vi "Filter SRs.vi"(8 "error in":errorcluster, 9 "Legend":refnum<vi>, 10 "Filter Cluster":T1={"Show Resolved"=TRUE, "Show Potentially Resolved"=TRUE, "Show Passoffs"=TRUE, "Show In Collab"=TRUE}, 11 "list in":T2[](array[typedef]) {"Creation Date" format="%<%x>T"; "Last Updated" format="%<%x>T"}) -> (0 "error out":errorcluster, 3 "list out":T2[](array[typedef]) {"Creation Date" format="%<%x>T"; "Last Updated" format="%<%x>T"})   [LabVIEW 2018]
uses:
  Type Defs/SR Cluster.ctl
  Type Defs/SR Status.ctl
  Type Defs/Filter Cluster.ctl
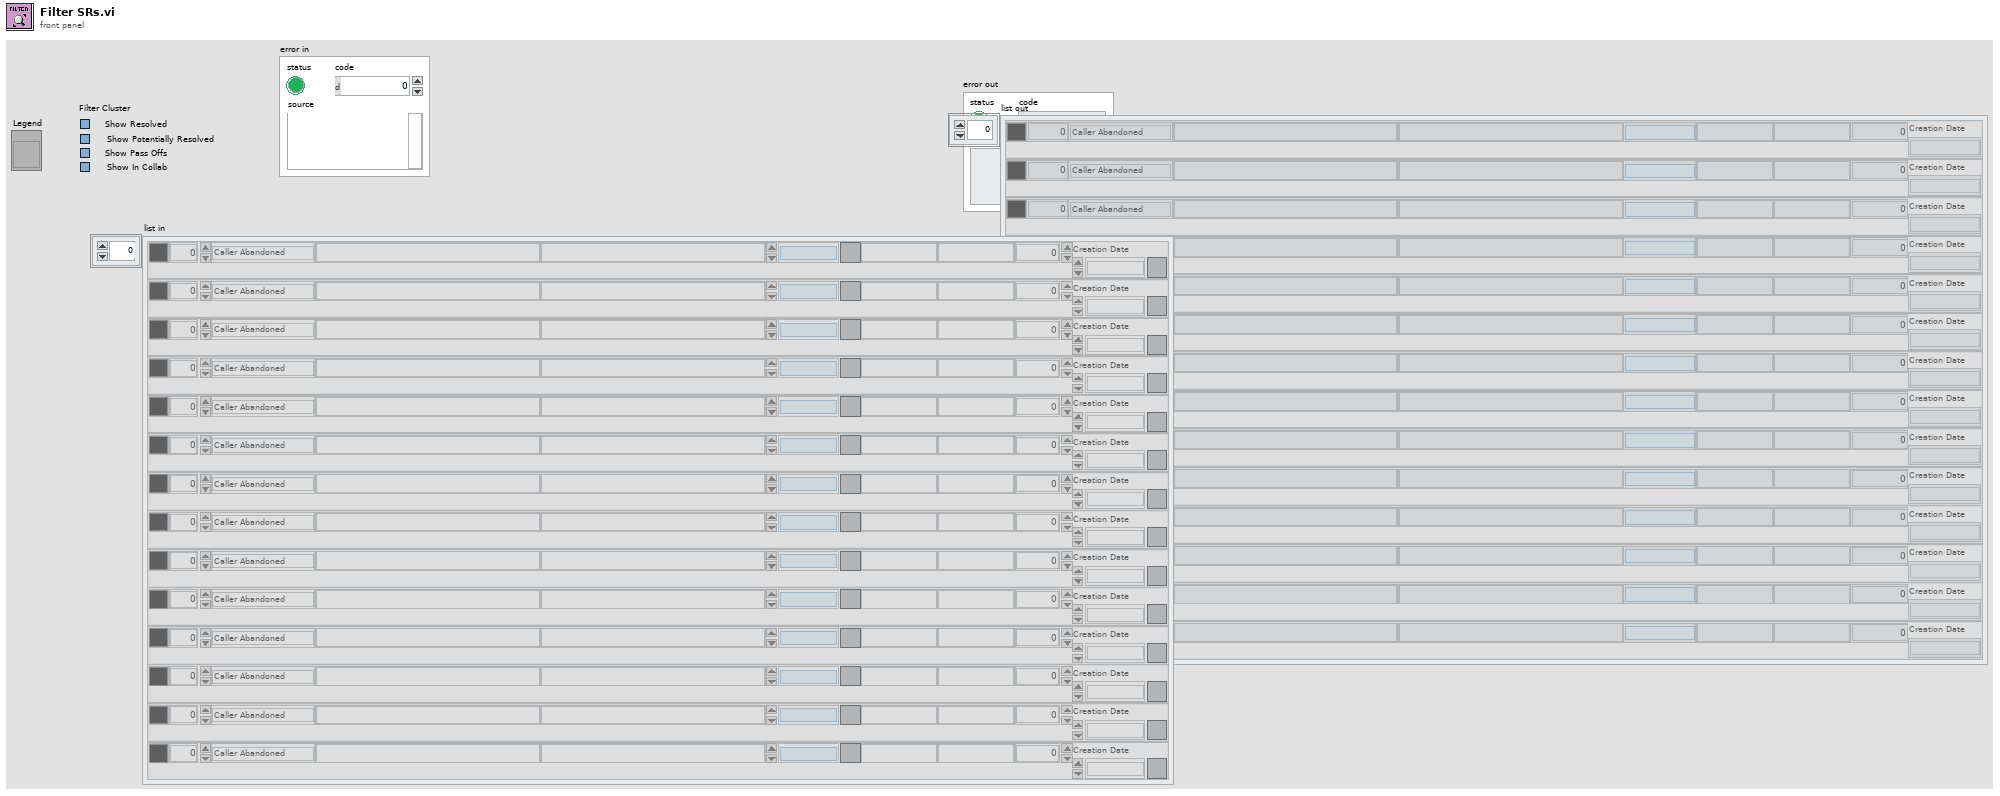
[diagram p1: front panel]
types:
  T1 = typedef "Filter Cluster.ctl" = cluster{"Show Resolved":bool, "Show Potentially Resolved":bool, "Show Passoffs":bool, "Show In Collab":bool}
  T2 = typedef "SR Cluster.ctl" = cluster{"Color":u32, "SR Number":i32, "SR Status":T3, "Name":string, "Summary":string, "Last Updated":timestamp, "SR Type":string, "Service Level":string, "Days Open":dbl, "Creation Date":timestamp}
  T3 = typedef "SR Status.ctl" = enum16{"Caller Abandoned", "Created in Error", "Expired", "Forum Resolved AE", "Forum Resolved Customer", "IN WORK", "IN WORK Collab with AES", "IN WORK Collab with PSE", "IN WORK Collab with SE", "IN WORK Customer Added Note", "IN WORK Escalation", "IN WORK Wait on Customer", "Open", "Potentially Resolved", "Presumed Resolved", "RMA Approved for Return", "RMA Closed", "RMA Closed - DOA", "RMA In Progress", "RMA Open", "RMA Waiting on Customer", "Resolved", "Passed Off"}
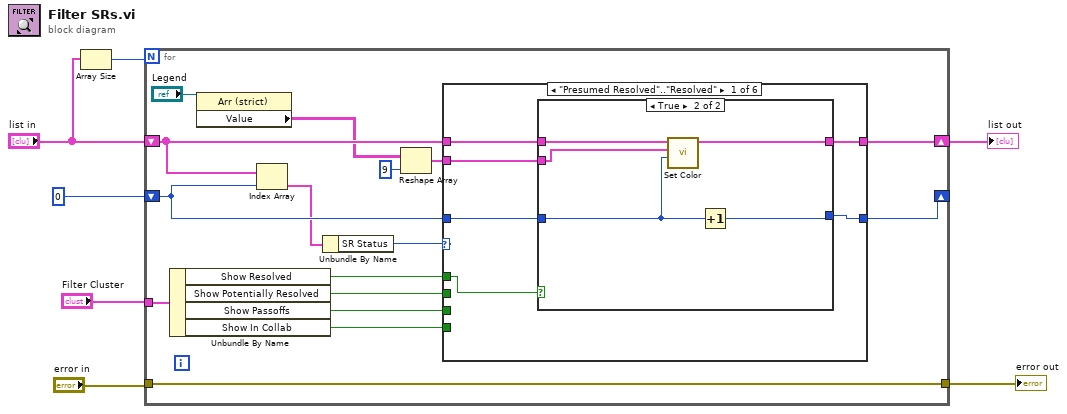
[diagram p0: block diagram]
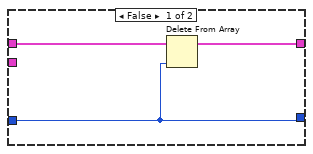
[diagram p2: hidden frame]
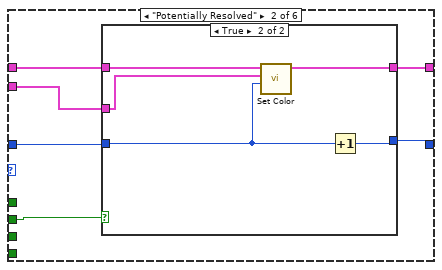
[diagram p3: hidden frame]
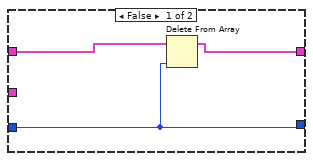
[diagram p4: hidden frame]
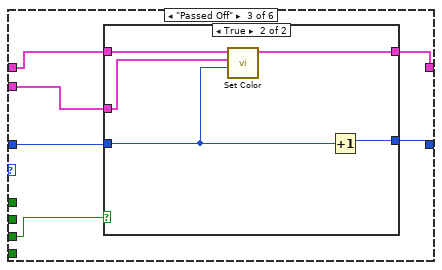
[diagram p5: hidden frame]
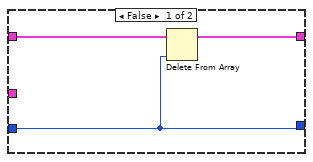
[diagram p6: hidden frame]
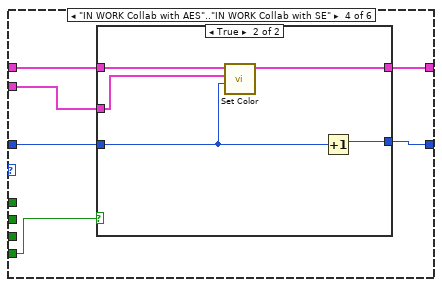
[diagram p7: hidden frame]
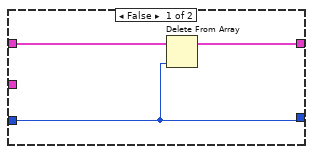
[diagram p8: hidden frame]
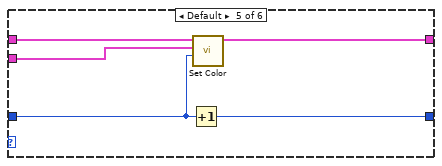
[diagram p9: hidden frame]
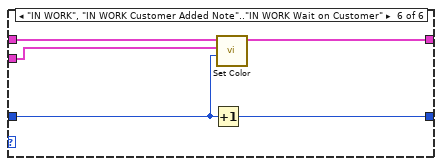
[diagram p10: hidden frame]
diagram:
  n1 = Array Size(array="list in") -> (size(s)=w6:i32)
  n2 = for {
    N: w6 -> [_]
    tunnel: "Filter Cluster" -> [w12]
    shift-right: [w16] -> w7
    shift-left: "list in" -> [w17]
    shift-right: [w18] -> _
    shift-left: 0 -> [w15]
    tunnel: "error in" -> [w14]
    tunnel: [w14] -> w3
    n3 = Unbundle By Name(w12) -> ("Show Resolved"=w22:bool, "Show Potentially Resolved"=w21:bool, "Show Passoffs"=w20:bool, "Show In Collab"=w19:bool)
    n4 = property class="Arr (strict)"(reference="Legend") -> ("Value"=w9:cluster{"Color Box":u32, "String":string}[][])  [unwired: 1 in, 2 out]
    n5 = Index Array(array=w17, index=w15) -> (element=w13:T2)
    n6 = Unbundle By Name(w13) -> ("SR Status"=w23:T3)
    n7 = Reshape Array(w9, 9 ("dimension size")) -> (w11:cluster{"Color Box":u32, "String":string}[])
    n8 = case shown="\"Presumed Resolved\"..\"Resolved\"" w23 {
      tunnel: w22 -> [w29 _ _ _ _ _]
      tunnel: w21 -> [_ w42 _ _ _ _]
      tunnel: w20 -> [_ _ w54 _ _ _]
      tunnel: w19 -> [_ _ _ w66 _ _]
      tunnel: w15 -> [w28 w43 w57 w71 w81 w86]
      tunnel: [w25 w41 w56 w70 w84 w87] -> w18
      tunnel: w17 -> [w27 w40 w52 w69 w83 w89]
      tunnel: [w26 w39 w55 w68 w82 w88] -> w16
      tunnel: w11 -> [w24 w38 w53 w67 w80 w85]
      frame "Presumed Resolved".."Resolved" {
        n9 = case shown="True" w29 {
          tunnel: w28 -> [w30 w35]
          tunnel: [w30 w34] -> w25
          tunnel: w27 -> [w32 w37]
          tunnel: [w31 w36] -> w26
          tunnel: w24 -> [_ w33]
          frame False {
            n10 = Delete From Array(array=w32, index=w30) -> (array with subset deleted=w31:T2[])  [unwired: 1 in, 1 out]
          }
          frame True {
            n11 = call "Set Color.vi"("index"=w35, "Flat Legend"=w33, "list in"=w37) -> ("list out"=w36:T2[])  [unwired: 8 in]
            n12 = Increment(x=w35) -> (x+1=w34:i32)
          }
        }
      }
      frame "Potentially Resolved" {
        n13 = case shown="True" w42 {
          tunnel: w43 -> [w44 w51]
          tunnel: [w44 w48] -> w41
          tunnel: w40 -> [w46 w50]
          tunnel: [w45 w49] -> w39
          tunnel: w38 -> [_ w47]
          frame False {
            n14 = Delete From Array(array=w46, index=w44) -> (array with subset deleted=w45:T2[])  [unwired: 1 in, 1 out]
          }
          frame True {
            n15 = call "Set Color.vi"("index"=w51, "Flat Legend"=w47, "list in"=w50) -> ("list out"=w49:T2[])  [unwired: 8 in]
            n16 = Increment(x=w51) -> (x+1=w48:i32)
          }
        }
      }
      frame "Passed Off" {
        n17 = case shown="True" w54 {
          tunnel: w57 -> [w58 w64]
          tunnel: [w58 w65] -> w56
          tunnel: w52 -> [w60 w63]
          tunnel: [w59 w62] -> w55
          tunnel: w53 -> [_ w61]
          frame False {
            n18 = Delete From Array(array=w60, index=w58) -> (array with subset deleted=w59:T2[])  [unwired: 1 in, 1 out]
          }
          frame True {
            n19 = call "Set Color.vi"("index"=w64, "Flat Legend"=w61, "list in"=w63) -> ("list out"=w62:T2[])  [unwired: 8 in]
            n20 = Increment(x=w64) -> (x+1=w65:i32)
          }
        }
      }
      frame "IN WORK Collab with AES".."IN WORK Collab with SE" {
        n21 = case shown="True" w66 {
          tunnel: w71 -> [w72 w76]
          tunnel: [w72 w79] -> w70
          tunnel: w69 -> [w74 w78]
          tunnel: [w73 w77] -> w68
          tunnel: w67 -> [_ w75]
          frame False {
            n22 = Delete From Array(array=w74, index=w72) -> (array with subset deleted=w73:T2[])  [unwired: 1 in, 1 out]
          }
          frame True {
            n23 = call "Set Color.vi"("index"=w76, "Flat Legend"=w75, "list in"=w78) -> ("list out"=w77:T2[])  [unwired: 8 in]
            n24 = Increment(x=w76) -> (x+1=w79:i32)
          }
        }
      }
      frame Default {
        n25 = Increment(x=w81) -> (x+1=w84:i32)
        n26 = call "Set Color.vi"("index"=w81, "Flat Legend"=w80, "list in"=w83) -> ("list out"=w82:T2[])  [unwired: 8 in]
      }
      frame "IN WORK", "IN WORK Customer Added Note".."IN WORK Wait on Customer" {
        n27 = Increment(x=w86) -> (x+1=w87:i32)
        n28 = call "Set Color.vi"("index"=w86, "Flat Legend"=w85, "list in"=w89) -> ("list out"=w88:T2[])  [unwired: 8 in]
      }
    }
  }
  "error out" <- w3
  "list out" <- w7
